vi "cv_08_01.vi"() -> ()   [LabVIEW 2013]
panel:
  out "Offset Past Match":i32
  out "Number Out":dbl
  out "String Length":u32
  out "Combined String":string
  in  "String 2":string="Volts DC:  +1.26E+1\r\n"
  in  "Trailer":string="Volts"
  in  "Numeric":dbl=6.0 format="%#_6f"
  in  "Header":string="The measurement is"
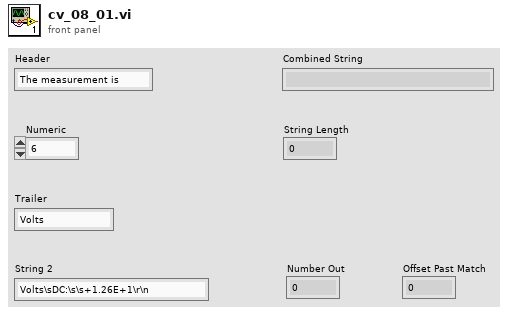
[diagram p1: front panel]
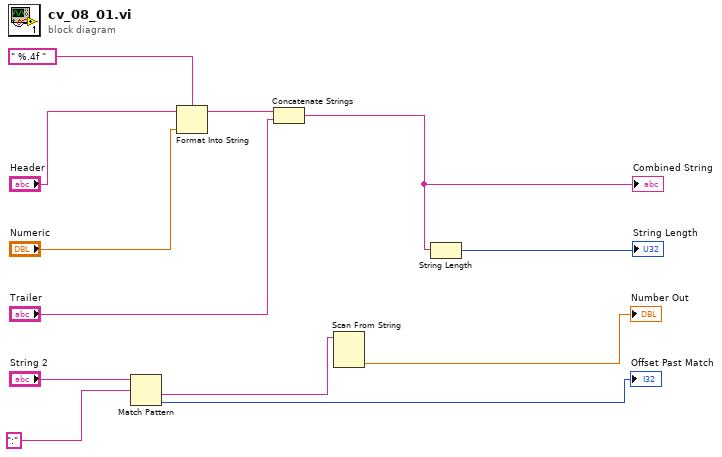
[diagram p0: block diagram]
diagram:
  n1 = Match Pattern(string="String 2", regular expression=":") -> (after substring=w2:string, offset past match=→"Offset Past Match":i32)  [unwired: 1 in, 2 out]
  n2 = Format Into String(format string=" %.4f ", initial string="Header", "Numeric") -> (resulting string=w9:string)  [unwired: 1 in, 1 out]
  n3 = Concatenate Strings(w9, "Trailer") -> (w6:string)
  "Combined String" <- w6
  n4 = Scan From String(input string=w2) -> (output 1=→"Number Out":dbl)  [unwired: 4 in, 3 out]
  n5 = String Length(string=w6) -> (length=→"String Length":i32)
